vi "190626_Simulation_AFTO2.vi"() -> ()   [LabVIEW 2019]
uses:
  <vilib>/Utility/Variable/NI_VariableUtilities.lvlib
panel:
  in  "X_eta":dbl=-50.0 format="%#_13g"
  in  "Z_eta":dbl=-50.0 format="%#_13g"
  out "q_out":dbl[][](array[numeric])
  in  "X_Type":string(combo)="Notch15"
  in  "Z_Type":string(combo)="Notch15"
  out "all time(s)":dbl
  out "Time slots (sec)":dbl[](array[numeric]) format="%#.10f"
  in  "Sample Rate (Hz)":dbl=1000.0 format="%#_13g"
  in  "STOP":bool
  in  "Load":bool
  in  "CLEAR":bool
  in  "RUN":bool
  out "RMS  X (um)":dbl format="%0.4f"
  out "MAX  X (um)":dbl format="%0.4f"
  out "RMS (one) X (um)":dbl format="%0.4f"
  out "Output X (mm)":dbl[](graph)
  out "CMD X (mm)":dbl[](graph)
  out "Position Error X (um)":dbl[](graph)
  out "Position Command X (mm)":dbl[](graph)
  out "time length":i32=15000
  out "start time":i32=7500
  out "RMS (one) Z (um)":dbl format="%0.4f"
  out "MAX  Z (um)":dbl format="%0.4f"
  out "RMS  Z (um)":dbl format="%0.4f"
  out "Position Error Z (um)":dbl[](graph)
  out "CMD Z (mm)":dbl[](graph)
  out "Output Z (mm)":dbl[](graph)
  out "Position Command Z (mm)":dbl[](graph)
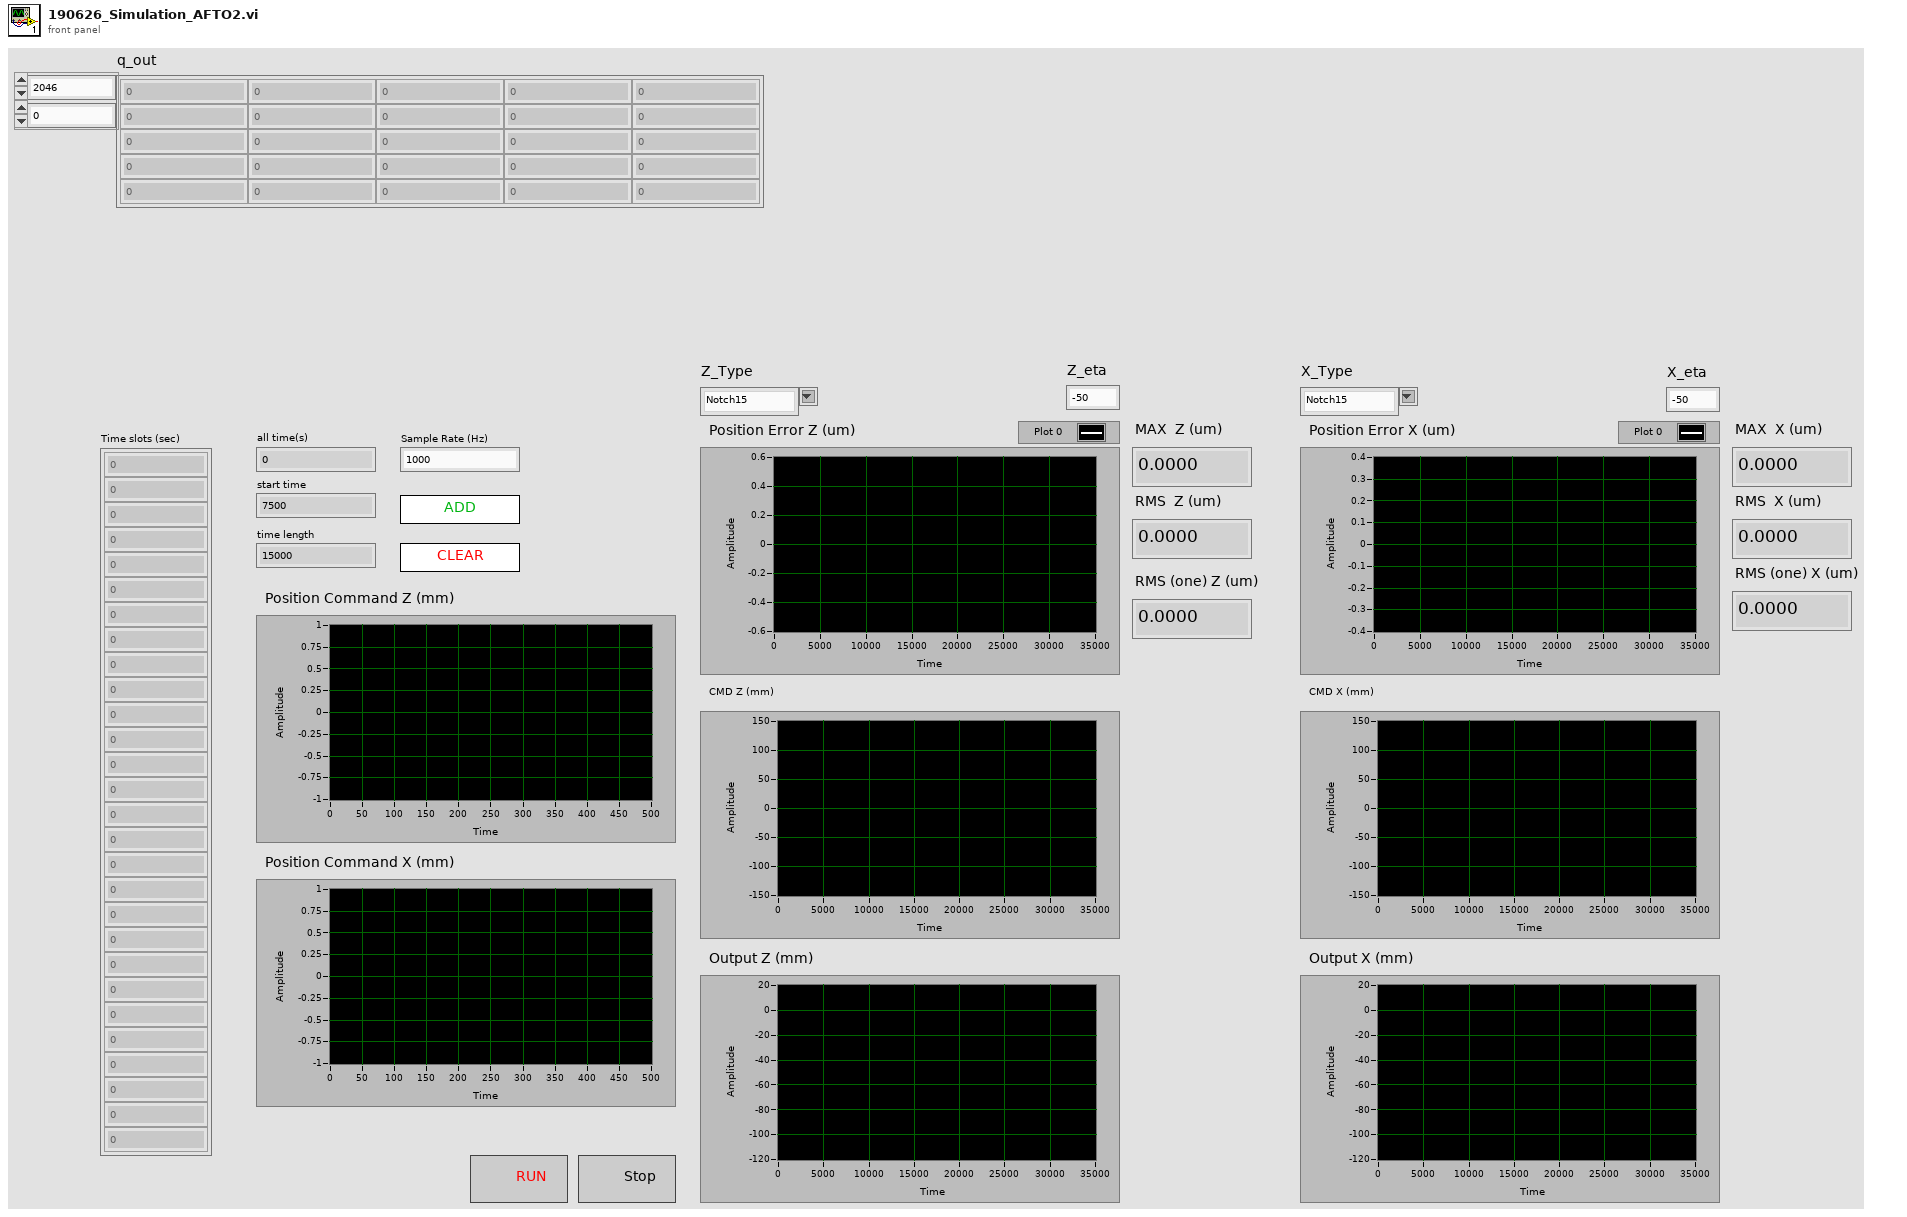
[diagram p1: front panel]
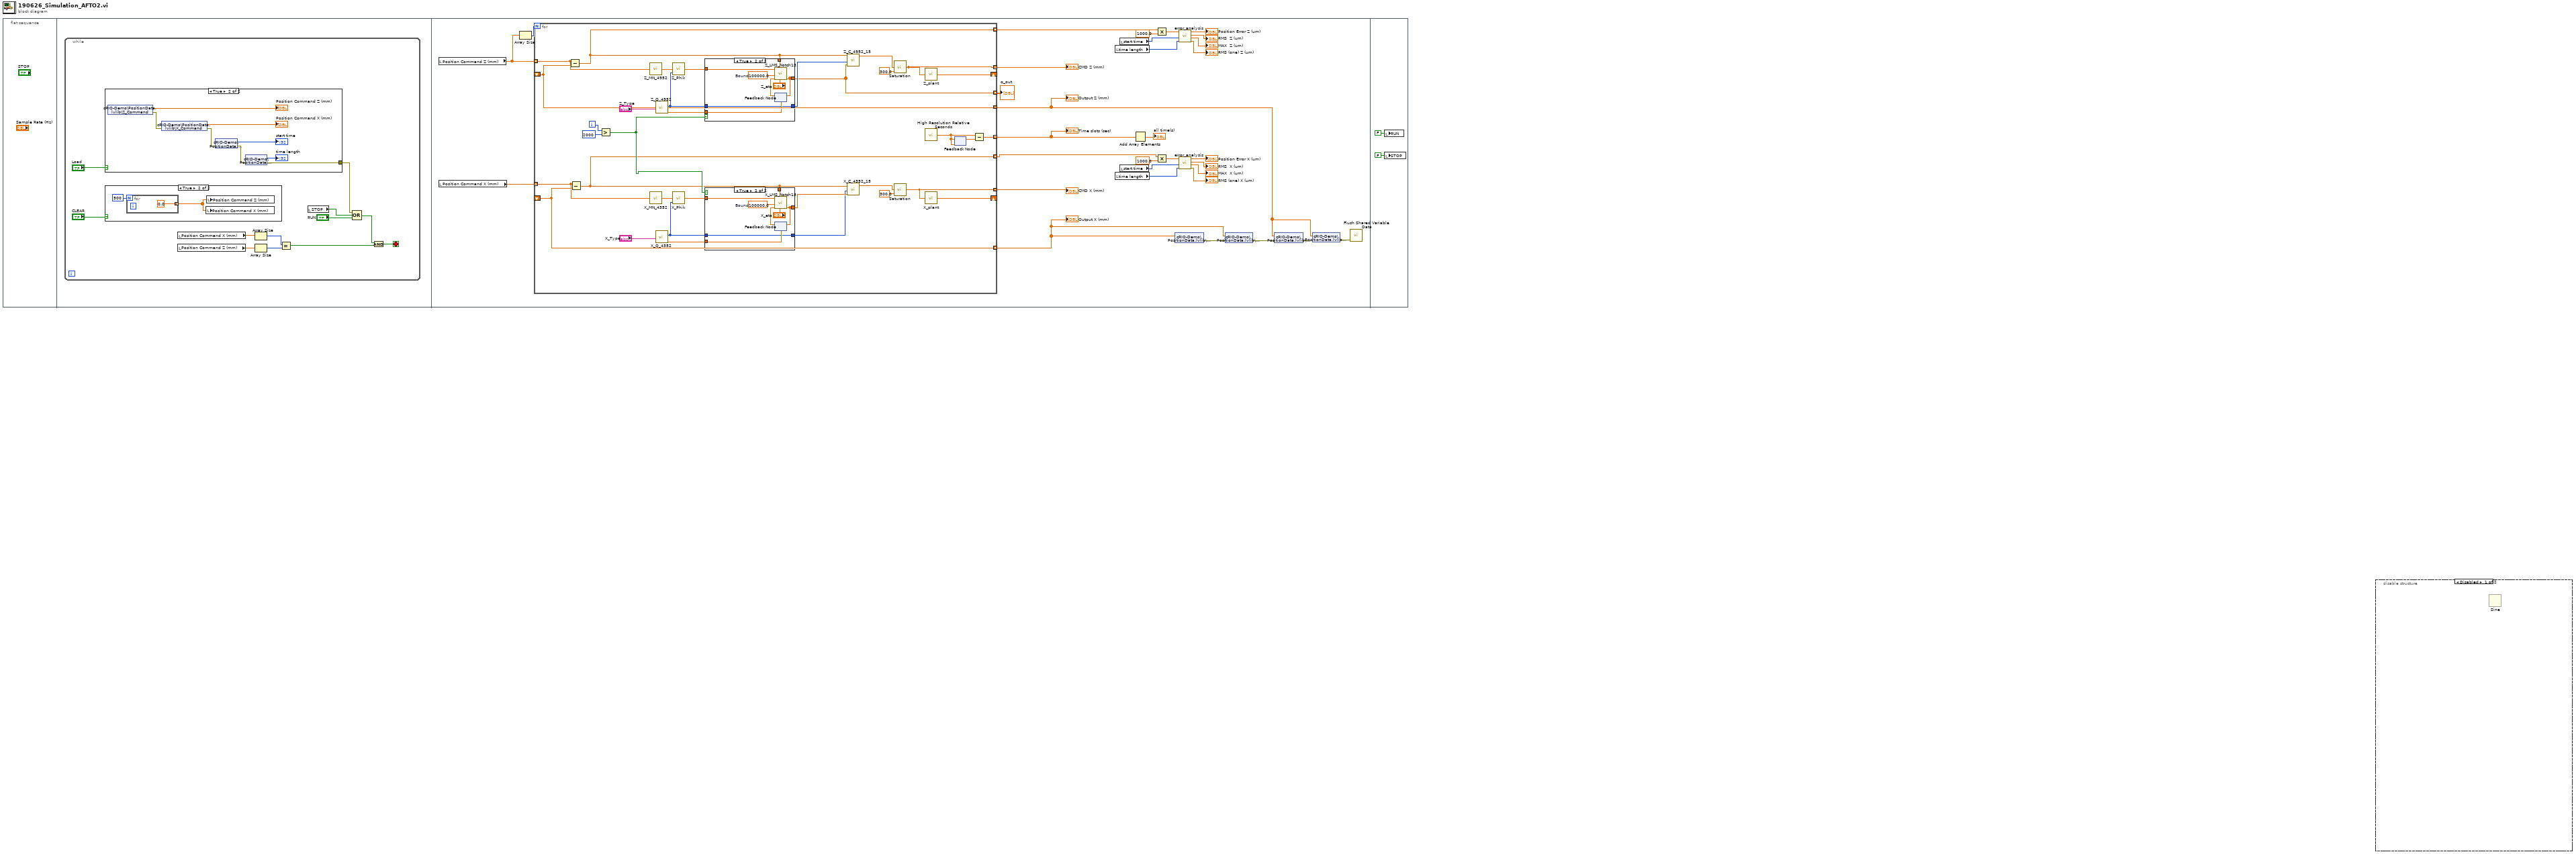
[diagram p0: block diagram]
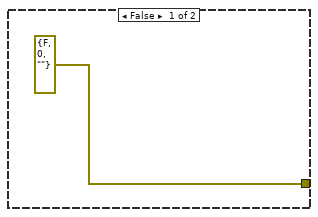
[diagram p3: hidden frame]
diagram:
  n1 = flat-sequence {
    frame #0 {
    }
    frame #1 {
      n2 = while {
        stop <- w9 stop-if-true
        n3 = case shown="True" "Load" {
          tunnel: [errorcluster {"status"=FALSE, "code"=0, "source"=""} ("error IO") w19] -> w1
          frame False {
          }
          frame True {
            n4 = shared-variable "cRIO-Demo\\PositionData.lvlib\\Z_Command"() -> (→"Position Command Z (mm)":dbl[], error out=w22:errorcluster)  [unwired: 1 in]
            n5 = shared-variable "cRIO-Demo\\PositionData.lvlib\\X_Command"(error in=w22) -> (→"Position Command X (mm)":dbl[], error out=w20:errorcluster)
            n6 = shared-variable "cRIO-Demo\\PositionData.lvlib\\t0"(error in=w20) -> (→"start time":i32, error out=w21:errorcluster)
            n7 = shared-variable "cRIO-Demo\\PositionData.lvlib\\tL"(error in=w21) -> (→"time length":i32, error out=w19:errorcluster)
          }
        }
        n8 = case shown="True" "CLEAR" {
          frame False {
          }
          frame True {
            n9 = for {
              N: 500 -> [_]
              tunnel: [0.0 ("element")] -> w14 mode=indexing
            }
            n10 = local write "Position Command X (mm)"(w14) -> ()
            n11 = local write "Position Command Z (mm)"(w14) -> ()
          }
        }
        n12 = local read "Position Command X (mm)"() -> (w10:dbl[])
        n13 = local read "Position Command Z (mm)"() -> (w11:dbl[])
        n14 = Array Size(array=w11) -> (size(s)=w7:i32)
        n15 = Array Size(array=w10) -> (size(s)=w8:i32)
        n16 = Equal?(x=w8, y=w7) -> (x = y?=w6:bool)
        n17 = local read "STOP"() -> (w2:bool)
        n18 = Compound Arithmetic op=OR(w1, w2, "RUN") -> (w4:bool)
        n19 = And(x=w4, y=w6) -> (x .and. y?=w9:bool)
      }
    }
    frame #2 {
      n20 = local read "Position Command Z (mm)"() -> (w55:dbl[])
      n21 = local read "Position Command X (mm)"() -> (w39:dbl[])
      n22 = Array Size(array=w55) -> (size(s)=w54:i32)
      n23 = for {
        N: w54 -> [_]
        shift-right: [w84] -> _
        shift-left: _ -> [w81]
        tunnel: [w81] -> w27 mode=indexing
        tunnel: [w69] -> w35 mode=indexing
        tunnel: [w83] -> w56 mode=indexing
        tunnel: w55 -> [w75] mode=indexing
        tunnel: w39 -> [w68] mode=indexing
        shift-right: [w85] -> _
        shift-left: _ -> [w80]
        tunnel: [w86] -> w38 mode=indexing
        tunnel: [w60] -> w33 mode=indexing
        tunnel: [w80] -> w28 mode=indexing
        tunnel: [w87] -> w37 mode=indexing
        tunnel: [w71] -> w25 mode=indexing
        i -> [w78]
        n24 = Subtract(x=w75, y=w81) -> (x-y=w69:dbl)
        n25 = Subtract(x=w68, y=w80) -> (x-y=w60:dbl)
        n26 = Greater?(x=w78, y=2000) -> (0:w65:bool)
        n27 = call "Z_MN_4952.vi"("u"=w75) -> ("y"=w76:dbl)  [unwired: 4 in]
        n28 = call "X_MN_4352.vi"("u"=w68) -> ("y"=w67:dbl)  [unwired: 4 in]
        n29 = call "Z_Q_4952.vi"("Type"="Z_Type") -> ("Qn"=w73:dbl[], "L"=w58:i32)  [unwired: 9 in]
        n30 = call "X_Q_4352.vi"("Type"="X_Type") -> ("Qn"=w59:dbl[], "L"=w57:i32)  [unwired: 9 in]
        n31 = call "Z_Phik.vi"("Lq"=w58, "u"=w76) -> ("phik"=w77:dbl[])  [unwired: 3 in]
        n32 = call "X_Phik.vi"("Lq"=w57, "u"=w67) -> ("phik"=w66:dbl[])  [unwired: 3 in]
        n33 = case shown="True" w65 {
          tunnel: w69 -> [_ w110]
          tunnel: w77 -> [_ w109]
          tunnel: [w101 w104] -> w71
          tunnel: w73 -> [w101 w106]
          tunnel: w58 -> [w102 w105]
          tunnel: [w102 w105] -> w72
          frame False {
          }
          frame True {
            w103 = 100000.0  # Bound
            n34 = feedback #1(w106) -> (w107:dbl[])
            n35 = call "Z_LMS_Notch15.vi"("eta"="Z_eta", "ek"=w110, "q_input"=w107, "Bound"=w103, "phik"=w109) -> ("q_out"=w104:dbl[])  [unwired: 4 in]
            n36 = feedback-in #1(w104) -> ()
          }
        }
        n37 = case shown="True" w65 {
          tunnel: w60 -> [_ w100]
          tunnel: w66 -> [_ w99]
          tunnel: [w91 w94] -> w64
          tunnel: w59 -> [w91 w96]
          tunnel: w57 -> [w92 w95]
          tunnel: [w92 w95] -> w63
          frame False {
          }
          frame True {
            w93 = 100000.0  # Bound
            n38 = feedback #2(w96) -> (w97:dbl[])
            n39 = call "X_LMS_Notch15.vi"("eta"="X_eta", "ek"=w100, "q_input"=w97, "Bound"=w93, "phik"=w99) -> ("q_out"=w94:dbl[])  [unwired: 4 in]
            n40 = feedback-in #2(w94) -> ()
          }
        }
        n41 = call "Z_C_4952_15.vi"("ek"=w69, "length"=w72, "q"=w71) -> ("uk"=w70:dbl)  [unwired: 4 in]
        n42 = call "X_C_4352_15.vi"("ek"=w60, "length"=w63, "q"=w64) -> ("uk"=w61:dbl)  [unwired: 4 in]
        n43 = call "Saturation.vi"("Vmax"=300.0, "uk"=w70) -> ("real uk"=w83:dbl)  [unwired: 3 in]
        n44 = call "Saturation.vi"("Vmax"=300.0, "uk"=w61) -> ("real uk"=w86:dbl)  [unwired: 3 in]
        n45 = call "Z_plant.vi"("u"=w83) -> ("y"=w84:dbl)  [unwired: 4 in]
        n46 = call <vilib>:"High Resolution Relative Seconds.vi"() -> ("relative seconds"=w82:dbl)
        n47 = call "X_plant.vi"("u"=w86) -> ("y"=w85:dbl)  [unwired: 4 in]
        n48 = feedback #3(w82) -> (w88:dbl)
        n49 = feedback-in #3(w82) -> ()
        n50 = Subtract(x=w82, y=w88) -> (x-y=w87:dbl)
      }
      "Output Z (mm)" <- w27
      "CMD Z (mm)" <- w56
      "Output X (mm)" <- w28
      "CMD X (mm)" <- w38
      "Time slots (sec)" <- w37
      "q_out" <- w25
      n51 = local read "time length"() -> (w49:i32)
      n52 = local read "time length"() -> (w43:i32)
      n53 = local read "start time"() -> (w48:i32)
      n54 = local read "start time"() -> (w42:i32)
      n55 = Add Array Elements(numeric array=w37) -> (sum=→"all time(s)":dbl)
      n56 = Multiply(x=w35, y=1000.0) -> (x*y=w47:dbl[])
      n57 = Multiply(x=w33, y=1000.0) -> (x*y=w40:dbl[])
      n58 = shared-variable "cRIO-Demo\\PositionData.lvlib\\X_EN"(w28) -> (error out=w30:errorcluster)  [unwired: 1 in]
      n59 = call "error_analysis.vi"("tLength"=w49, "t0"=w48, "data in (um)"=w47) -> ("rms (one) (um)"=→"RMS (one) Z (um)":dbl, "max err (um)"=→"MAX  Z (um)":dbl, "rms (all) (um)"=→"RMS  Z (um)":dbl, "data out (um)"=→"Position Error Z (um)":dbl[])  [unwired: 5 in]
      n60 = call "error_analysis.vi"("tLength"=w43, "t0"=w42, "data in (um)"=w40) -> ("rms (one) (um)"=→"RMS (one) X (um)":dbl, "max err (um)"=→"MAX  X (um)":dbl, "rms (all) (um)"=→"RMS  X (um)":dbl, "data out (um)"=→"Position Error X (um)":dbl[])  [unwired: 5 in]
      n61 = shared-variable "cRIO-Demo\\PositionData.lvlib\\X_LS"(w28, error in=w30) -> (error out=w29:errorcluster)
      n62 = shared-variable "cRIO-Demo\\PositionData.lvlib\\Z_EN"(w27, error in=w29) -> (error out=w31:errorcluster)
      n63 = shared-variable "cRIO-Demo\\PositionData.lvlib\\Z_LS"(w27, error in=w31) -> (error out=w26:errorcluster)
      n64 = call <vilib>:"Flush Shared Variable Data.vi"("error in (no error)"=w26) -> ()  [unwired: 10 in, 1 out]
    }
    frame #3 {
      n65 = local write "RUN"(FALSE ("RUN")) -> ()
      n66 = local write "STOP"(FALSE ("STOP")) -> ()
    }
  }
  n67 = disable-structure shown="Disabled" {
    frame Disabled {
      n68 = Sine() -> ()  [unwired: 1 in, 1 out]
    }
    frame Enabled {
    }
  }
